vi "NF87XX.get position.vi"(0 "i ref in":refnum<vi>, 5 "error in (no error)":errorcluster) -> (14 "i ref out":refnum<vi>, 17 "Positions":i32[](array[numeric]), 19 "error out":errorcluster)   [LabVIEW 2014, in "NF87XX.lvlib"]
doc: "Returns the positions of the systems.\n\n\nauthor: Stefan Götte\ndata: 09-JAN-2007\n\n\nLicense Agreement for this software:\n\nCopyright (C)\nGesellschaft für Schwerionenforschung, GSI\nPlanckstr. 1\n64291 Darmstadt\nGermany\n\nContact: D.Beck@gsi.de \n\nThis program is free software; you can redistribute it and/or modify it under the terms of the GNU General Public License as published by the Free Software Foundation; either version 2 of the license, or (at your option) any later version.\n\nThis program is distributed in the hope that it will be useful, but WITHOUT ANY WARRANTY; without even the implied warranty of MERCHANTABILITY or FITNESS FOR A PARTICULAR PURPOSE. See the GNU General License for more details (http://www.gnu.org).\n\nGesellschaft für Schwerionenforschung, GSI\nPlanckstr. 1, 64291 Darmstadt, Germany\nFor all questions and ideas contact: M.Richter@gsi.de, H.Brand@gsi.de or D.Beck@gsi.de.\nLast update: 17-JUN-2004"
uses:
  NF87XX.lvlib
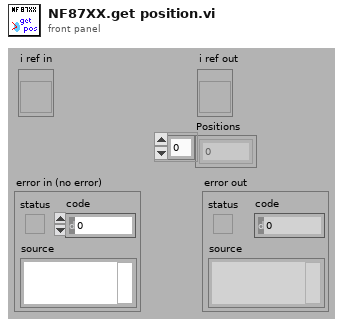
[diagram p1: front panel]
types:
  T1 = enum16{"User....", "DEF", "DIAG", "INI", "LOCK", "UNLOCK", "MAP", "SAV", "VER", "ACC", "CHL", "FOR", "GO", "HAL", "MOF", "MON", "MPV", "POS", "REL", "REV", "STA", "STO", "TYP", "VEL", "ABS", "SER", "NOS", "DRT", "FLI", "RLI", "FIN", "RIN", "AIN", "IN", "JOF", "JON", "OUT", "RES FINE", "RES COARSE", "02 (HEX)", "PWM", "CNT", "TMR", "HOSTNAME", "IPADDR", "IPMODE", "NETMASK", "GATEWAY", "DNSSRVR", "PASSWD", "ECHO", "MACADDR"}
  T2 = typedef "NF87XX.lvlib/NF87XX.i attribute.ctl" = cluster{"Con Settings":T3, "Drivers":T4[], "Status":cluster{"Service ID":i32, "Status":T7}, "Joystick available":bool, "VISA Resource":string}
  T3 = typedef "NewFocusPico - Driver np.lvlib/VISA & TCPIP Control.ctl" = cluster{"VISA or TCP/IP":bool, "Init Connection":bool, "Close Connection":bool, "Resource Name":refnum<visa-resource-name>, "hostname":string, "connection ID":refnum<k5>}
  T4 = typedef "NF87XX.lvlib/NF87XX.driver Settings.ctl" = cluster{"Name":string, "Driver Type":T5, "Pico Parameter type":T6, "Acceleration [Steps/s²]":cluster{"Motor 0":dbl, "Motor 1":dbl, "Motor 2":dbl}, "Start Velocity [Steps/s]":cluster{"Motor 0":dbl, "Motor 1":dbl, "Motor 2":dbl}, "Velocity [Steps/s]":cluster{"Motor 0":dbl, "Motor 1":dbl, "Motor 2":dbl}, "axis channel":i32, "Position":i32, "Position Service ID":i32}
  T5 = typedef "NF87XX.lvlib/NF87XX.driver Type.ctl" = enum16{"not defined", "3-ch open loop drv", "1-ch closed loop drv"}
  T6 = typedef "NewFocusPico - Driver np.lvlib/Pico Parameters.ctl" = cluster{"Pico Type":enum16{"Open-Loop Pico", "Close-Loop Pico", "Pico Ultra"}, "Acceleration (steps/sec^2)":string, "Velocity ( Hz)":string, "Driver":string, "Motor":string, "Channel":string, "Process Step":string}
  T7 = typedef "PH_StatusHandler.lvlib/PH_StatusHandler.Status.ctl" = i16
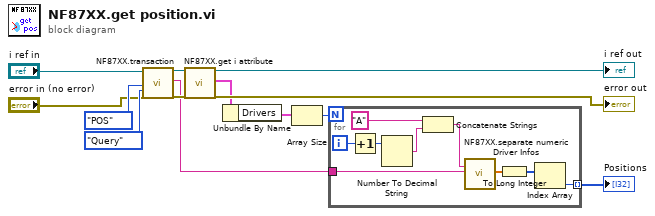
[diagram p0: block diagram]
diagram:
  n1 = call "NF87XX.transaction.vi"("i ref in"="i ref in", "MCL Cmd"=T1."POS", "Query/Set"=enum16{"Query", "Set"}."Query", "error in (no error)"="error in (no error)") -> ("i ref out"=w9:refnum<vi>, "Read String"=w2:string, "error out"=w7:errorcluster)  [unwired: 13 in]
  n2 = call "NF87XX.get i attribute.vi"("i ref in"=w9, "error in (no error)"=w7) -> ("i ref out"=→"i ref out":refnum<vi>, "i attribute"=w5:T2, "error out"=→"error out":errorcluster)  [unwired: 15 in]
  n3 = Unbundle By Name(w5) -> ("Drivers"=w4:T4[])
  n4 = Array Size(array=w4) -> (size(s)=w3:i32)
  n5 = for {
    N: w3 -> [_]
    tunnel: w2 -> [w22]
    tunnel: [w18] -> w1 mode=indexing
    i -> [w20]
    n6 = Increment(x=w20) -> (x+1=w19:i32)
    n7 = Number To Decimal String(number=w19) -> (decimal integer string=w17:string)  [unwired: 1 in]
    n8 = Concatenate Strings("A", w17) -> (w16:string)
    n9 = call "NF87XX.separate numeric Driver Infos.vi"("Driver"=w16, "Read String"=w22) -> ("Result"=w15:dbl[])  [unwired: 17 in]
    n10 = To Long Integer(number=w15) -> (32bit integer=w14:i32[])
    n11 = Index Array(array=w14) -> (element=w18:i32)  [unwired: 1 in]
  }
  "Positions" <- w1
